vi "Setpoint current control.vi"(8 "error in":errorcluster, 10 "setpoint":dbl=20.0 format="%.2f", 11 "Meerstetter Lib.lvlib:TEC 1090":refnum<class "Meerstetter TEC.lvclass">) -> (0 "error out":errorcluster, 3 "TEC 1090 out":refnum<class "Meerstetter TEC.lvclass">)   [LabVIEW 2014, in "Meerstetter Lib.lvlib" / "Meerstetter TEC.lvclass"]
uses:
  Meerstetter TEC.lvclass
  Generic TEC/TEC.lvclass/TEC.ctl
  <vilib>/addons/control/pid/pid.llb/PID (DBL).vi
  Generic TEC/TEC.lvclass
  <vilib>/addons/control/pid/NI_PID_pid.lvlib
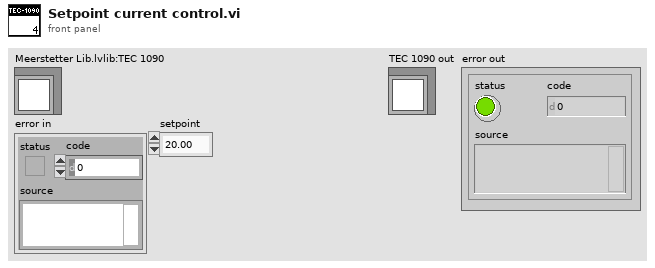
[diagram p1: front panel]
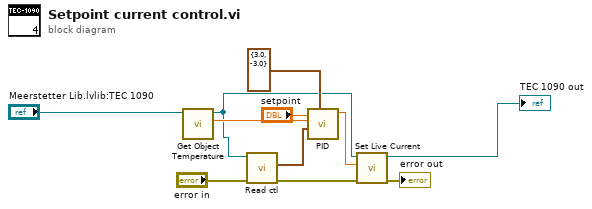
[diagram p0: block diagram]
diagram:
  n1 = call "Get Object Temperature.vi"("TEC 1090 in"="Meerstetter Lib.lvlib:TEC 1090") -> ("Number"=w5:sgl, "TEC 1090 out"=w1:refnum<class "Meerstetter TEC.lvclass">)  [unwired: 8 in, 1 out]
  n2 = call "Read ctl.vi"("error in (no error)"="error in", "TEC in"=w1) -> ("error out"=w8:errorcluster, "ctl"=w11:cluster{"p":dbl, "i":dbl, "d":dbl})  [unwired: 7 in, 1 out]
  n3 = call-poly <vilib>:"PID.vi"("output range"=cluster{"output high":dbl, "output low":dbl} {"output high"=3.0, "output low"=-3.0}, "PID gains"=w11, "process variable"=w5, "setpoint"="setpoint") -> ("output"=w10:dbl)  [unwired: 6 in, 1 out]
  n4 = call "Set Live Current.vi"("error in"=w8, "I"=w10, "TEC 1090 in"=w1) -> ("error out"=→"error out":errorcluster, "TEC 1090 out"=→"TEC 1090 out":refnum<class "Meerstetter TEC.lvclass">)  [unwired: 7 in]
